vi "send_common_trigger.vi"(8 "error in (no error)":errorcluster, 10 "trigger":T1, 11 "GenericExperiment in":refnum<class "ExperimentControllerDL090430DAQmxTriggered.lvclass">) -> (0 "error out":errorcluster, 3 "GenericExperiment out":refnum<class "ExperimentControllerDL090430DAQmxTriggered.lvclass">, 4 "# elements in queue":i32)   [LabVIEW 2010, in "ExperimentControllerDL090430DAQmxTriggered.lvclass"]
uses:
  ExperimentControllerDL090430DAQmxTriggered.lvclass
  common/classes/GenericToplevelComponent/GenericToplevelComponent/common_trigger_enum.ctl
  GenericExperimentController/GenericExperimentController/GenericExperimentController.lvclass
  ExperimentControllerDL090430DAQmxTriggered.lvclass/ExperimentControllerDL090430DAQmxTriggered.ctl
  common/classes/GenericToplevelComponent/GenericToplevelComponent/GenericToplevelComponent.lvclass
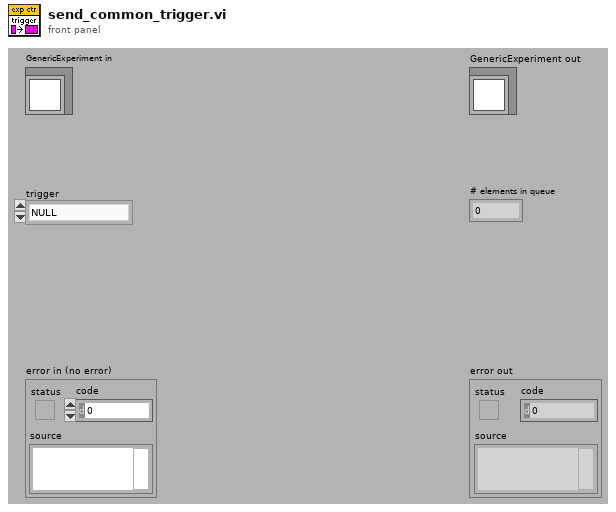
[diagram p1: front panel]
types:
  T1 = typedef "GenericToplevelComponent.lvclass/common_trigger_enum.ctl" = enum16{"NULL", "initialise", "terminate", "fetch command", "fetch data", "attach observer", "register as observer", "detach observer", "acknowledge", "start", "stop"}
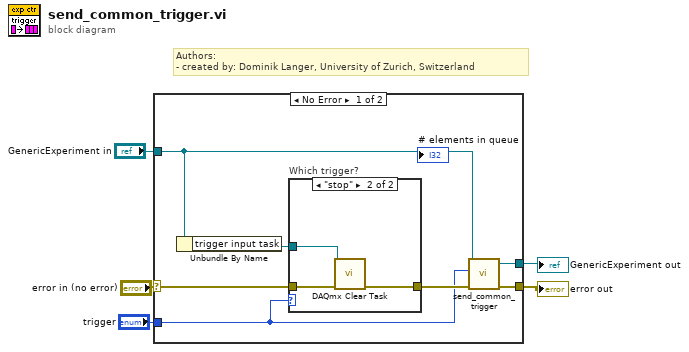
[diagram p0: block diagram]
diagram:
  # "Authors: \n- created by: Dominik Langer, University of Zurich, Switzerland"
  n1 = case shown="No Error" "error in (no error)" {
    selector: "error in (no error)" -> [w12 w17]
    tunnel: "trigger" -> [w6 _]
    tunnel: "GenericExperiment in" -> [w7 w18]
    tunnel: [w8 w18] -> w2
    tunnel: [w9 w17] -> w1
    frame No Error {
      n2 = Unbundle By Name(w7) -> ("trigger input task"=w11:refnum<k21>)
      n3 = case "Which trigger?" shown="\"stop\"" w6 {
        tunnel: w11 -> [_ w14]
        tunnel: w12 -> [w13 w16]
        tunnel: [w13 w15] -> w10
        frame Default {
        }
        frame "stop" {
          n4 = call <vilib>:"DAQmx Clear Task.vi"("task in"=w14, "error in"=w16) -> ("error out"=w15:errorcluster)  [unwired: 13 out]
        }
      }
      n5 = call-parent "send_common_trigger.vi"("error in (no error)"=w10, "trigger"=w6, "GenericToplevelComponent in"=w7) -> ("error out"=w9:errorcluster, "GenericToplevelComponent out"=w8:refnum<class "ExperimentControllerDL090430DAQmxTriggered.lvclass">)  [unwired: 6 in, 1 out]
    }
    frame Error {
    }
  }
  "error out" <- w1
  "GenericExperiment out" <- w2
